vi "Pre Launch Init.vi"(11 "Nested in":refnum<class "Home.lvclass">) -> (0 "error out":errorcluster, 3 "Nested out":refnum<class "Home.lvclass">)   [LabVIEW 2024, in "Home.lvlib" / "Home.lvclass"]
doc: "(<B>Filename</B>: Actor Framework.lvlib:Actor.lvclass:Pre Launch Init.vi)\n\nDefines behavior that occurs after the Launch Nested Actor method is invoked but before the actor's Actor Core method begins running.\n\nBy default, this method does nothing. A descendant class may override it to define behavior."
uses:
  Home.lvclass
  Home.lvclass/Home.ctl
  <vilib>/MGI/Panel Manager/Panel Actor/Panel Actor/Panel Actor.lvclass
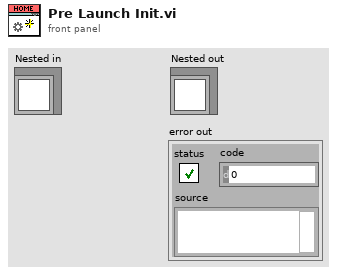
[diagram p1: front panel]
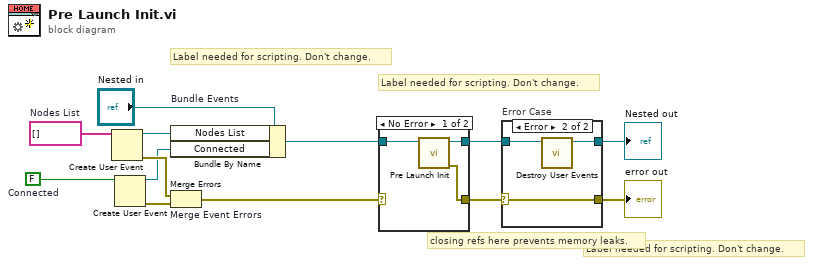
[diagram p0: block diagram]
diagram:
  w3 = FALSE  # Connected
  w5 = string[] []  # Nodes List
  # "Label needed for scripting. Don't change."
  # "Label needed for scripting. Don't change."
  # "Label needed for scripting. Don't change."
  # "closing refs here prevents memory leaks."
  n1 = Create User Event(user event datatype=w5) -> (user event=w4:refnum<user-event>, error out=w12:errorcluster)  [unwired: 1 in]
  n2 = Create User Event(user event datatype=w3) -> (user event=w2:refnum<user-event>, error out=w1:errorcluster)  [unwired: 1 in]
  n3 = Bundle By Name "Bundle Events"(cluster="Nested in", "Nodes List"=w4, "Connected"=w2) -> (w8:refnum<class "Home.lvclass">)
  n4 = Merge Errors "Merge Event Errors"(w12, w1) -> (w7:errorcluster)
  n5 = case shown="No Error" w7 {
    selector: w7 -> [_ w18]
    tunnel: [w16 w17] -> w9
    tunnel: w8 -> [w15 w17]
    tunnel: [w14 w18] -> w6
    frame No Error {
      n6 = call-parent "Pre Launch Init.vi"("Panel Actor in"=w15) -> ("error out"=w14:errorcluster, "Panel Actor out"=w16:refnum<class "Home.lvclass">)  [unwired: 9 in]
    }
    frame Error {
    }
  }
  n7 = case "Error Case" shown="Error" w6 {
    selector: w6 -> [w19 w23]
    tunnel: w9 -> [w20 w22]
    tunnel: [w20 w21] -> w11
    tunnel: [w19 w23] -> w10
    frame No Error {
    }
    frame Error {
      n8 = call "Destroy User Events.vi"("UI Template in"=w22) -> ("UI Template out"=w21:refnum<class "Home.lvclass">)  [unwired: 10 in]
    }
  }
  "error out" <- w10
  "Nested out" <- w11
